vi "Close.vi"(8 "Error In":errorcluster, 11 "XBMC Ref":T1) -> (0 "Error Out":errorcluster)   [LabVIEW 2013, in "LVH-XBMC.lvlib"]
uses:
  LVH-XBMC.lvlib
  Private/Type Defs/XBMC Ref.ctl
  <vilib>/httpClient/ClientHandle.ctl
  <vilib>/httpClient/LabVIEWHTTPClient.lvlib
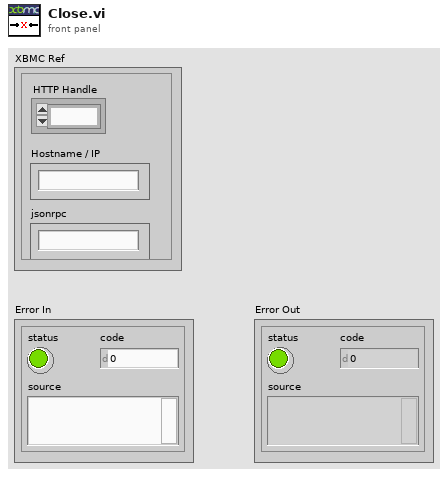
[diagram p1: front panel]
types:
  T1 = typedef "LVH-XBMC.lvlib/XBMC Ref.ctl" = cluster{"HTTP Handle":T2, "Hostname / IP":string, "jsonrpc":string}
  T2 = typedef "LabVIEWHTTPClient.lvlib/ClientHandle.ctl" = refnum<k1>
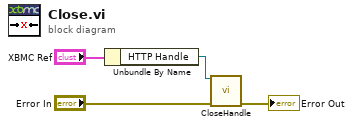
[diagram p0: block diagram]
diagram:
  n1 = Unbundle By Name("XBMC Ref") -> ("HTTP Handle"=w3:T2)
  n2 = call <vilib>:"CloseHandle.vi"("client handle"=w3, "error in (no error)"="Error In") -> ("error out"=→"Error Out":errorcluster)  [unwired: 13 in]
